vi "mass_damper.vi"(6 "dt":dbl=1.0 format="%0.2f", 7 "Reset":bool, 8 "B":dbl, 9 "Mass":dbl=1.0 format="%#_13g", 11 "f(t)":dbl) -> (1 "x_ddot(t)":dbl format="%0.2f", 2 "x_dot(t)":dbl format="%0.2f", 3 "x(t)":dbl format="%0.2f")   [LabVIEW 2014]
uses:
  <vilib>/ptbypt/NI_PtbyPt.lvlib
panel:
  # "Simulate a mass with damping\nInput: force\noutput: x, x_dot, x_dot_dot"
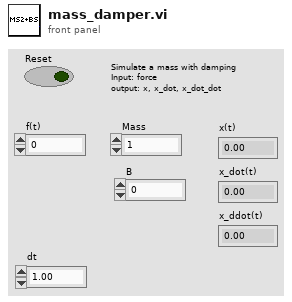
[diagram p1: front panel]
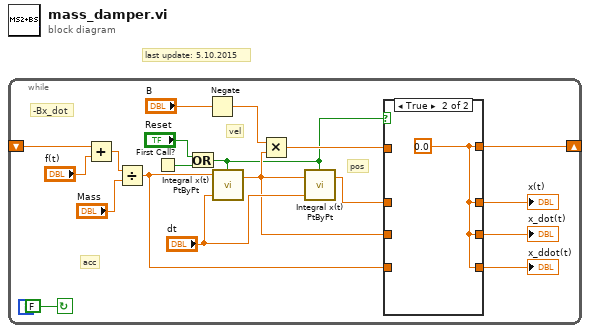
[diagram p0: block diagram]
diagram:
  # "last update: 5.10.2015"
  n1 = while {
    shift-right: [w14] -> _
    shift-left: _ -> [w15]
    stop <- FALSE continue-if-true
    # "pos"
    # "vel"
    # "acc"
    # "-Bx_dot"
    n2 = Add(x=w15, y="f(t)") -> (x+y=w4:dbl)
    n3 = Divide(x=w4, y="Mass") -> (x/y=w5:dbl)
    n4 = First Call?() -> (First Call?: T/F=w2:bool)
    n5 = Or(x="Reset", y=w2) -> (x .or. y?=w6:bool)
    n6 = Negate(x="B") -> (-x=w16:dbl)
    n7 = call <vilib>:"Integral x(t) PtByPt.vi"("initialize"=w6, "dt"="dt", "x"=w5) -> ("integral x(t)"=w7:dbl)  [unwired: 1 in, 1 out]
    n8 = Multiply(x=w16, y=w7) -> (x*y=w13:dbl)
    n9 = call <vilib>:"Integral x(t) PtByPt.vi"("initialize"=w6, "dt"="dt", "x"=w7) -> ("integral x(t)"=w8:dbl)  [unwired: 1 in, 1 out]
    n10 = case shown="True" w6 {
      tunnel: [w23 w24] -> w14
      tunnel: w13 -> [w23 _]
      tunnel: [w22 w24] -> w12
      tunnel: w7 -> [w22 _]
      tunnel: [w21 w24] -> w11
      tunnel: w8 -> [w21 _]
      tunnel: [w20 w24] -> w10
      tunnel: w5 -> [w20 _]
      frame False {
      }
      frame True {
        w24 = 0.0
      }
    }
    "x(t)" <- w11
    "x_dot(t)" <- w12
    "x_ddot(t)" <- w10
  }
